vi "Write Test Value.vi"(8 "error in (no error)":errorcluster, 10 "Value":dbl, 11 "Test in":refnum<class "Test.lvclass">) -> (0 "error out":errorcluster, 3 "Test out":refnum<class "Test.lvclass">)   [LabVIEW 2014, in "Test.lvclass"]
uses:
  Test.lvclass
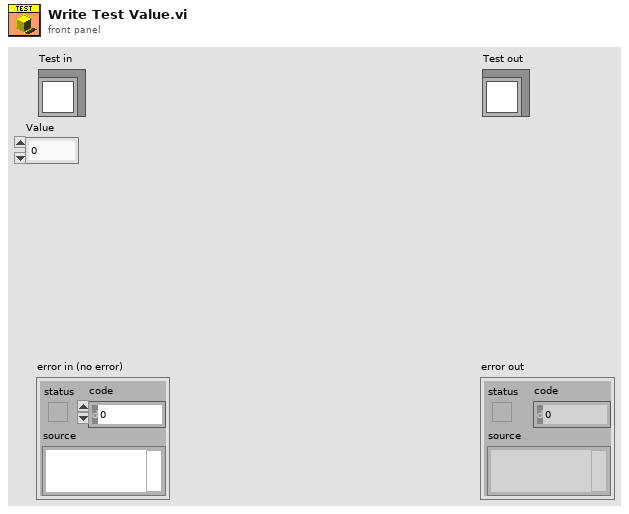
[diagram p1: front panel]
types:
  T1 = typedef "Test.lvclass/ObjectAttributes.ctl" = cluster{"Value":dbl}
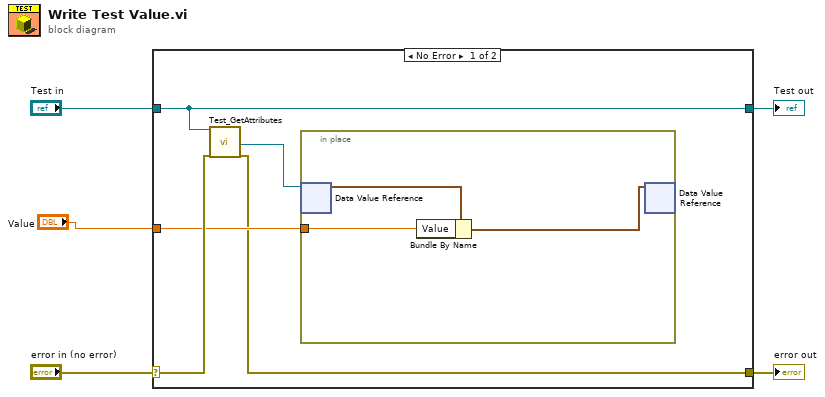
[diagram p0: block diagram]
diagram:
  n1 = case shown="No Error" "error in (no error)" {
    selector: "error in (no error)" -> [w9 w15]
    tunnel: [w6 w15] -> w4
    tunnel: [w10 w14] -> w2
    tunnel: "Test in" -> [w10 w14]
    tunnel: "Value" -> [w7 _]
    frame No Error {
      n2 = call "Test_GetAttributes.vi"("reference in"=w10, "error in (no error)"=w9) -> ("DataRef"=w8:refnum<data-value>, "error out"=w6:errorcluster)  [unwired: 14 in, 2 out]
      n3 = in-place {
        in-place-border: w7 -> [w11]
        n4 = in-place-dvr #1(w8) -> (w13:T1)  [unwired: 1 out]
        n5 = Bundle By Name(cluster=w13, "Value"=w11) -> (w12:T1)
        n6 = in-place-dvr #1(w12) -> ()  [unwired: 2 out]
      }
    }
    frame Error {
    }
  }
  "error out" <- w4
  "Test out" <- w2
